vi "createChildEvents.vi"(8 "error in (no error)":errorcluster, 11 "SettingsEventsManager in":refnum<class "SettingsEventsManager.lvclass">) -> (0 "error out":errorcluster, 3 "SettingsEventsManager out":refnum<class "SettingsEventsManager.lvclass">)   [LabVIEW 2009, in "Tools.lvlib" / "Settings.lvlib" / "SettingsEventsManager.lvclass"]
uses:
  SettingsEventsManager.lvclass
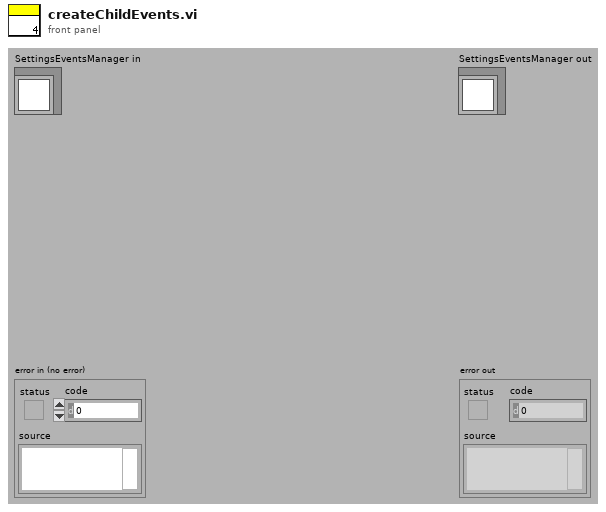
[diagram p1: front panel]
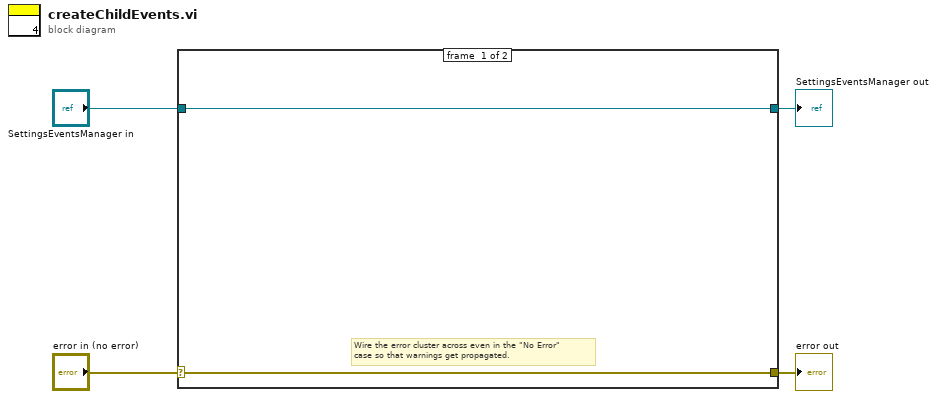
[diagram p0: block diagram]
diagram:
  n1 = case shown="No Error" "error in (no error)" {
    selector: "error in (no error)" -> [w5 w8]
    tunnel: [w5 w8] -> w3
    tunnel: [w6 w7] -> w1
    tunnel: "SettingsEventsManager in" -> [w6 w7]
    frame #0 {
      # "Wire the error cluster across even in the \"No Error\"\ncase so that warnings get propagated."
    }
    frame #1 {
    }
  }
  "error out" <- w3
  "SettingsEventsManager out" <- w1
